vi "Initialise.vi"   [LabVIEW 2020, in "RTAF.lvlib"]
uses:
  RTAF.lvlib
  Actors/Alarms Handler/API/Alarms Handler Actor API.lvclass
  Actors/Logger/API/Logger Actor API.lvclass
  Actors/System Status/API/System Status Actor API.lvclass
  Actors/Test/API/Test Actor API.lvclass
  Actors/Global References.vi
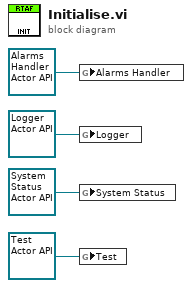
[diagram p0: block diagram]
diagram:
  n1 = global write "Global References.vi" "Alarms Handler"(refnum<class "Alarms Handler Actor API.lvclass"> refnum ("Alarms Handler")) -> ()
  n2 = global write "Global References.vi" "Logger"(refnum<class "Logger Actor API.lvclass"> refnum ("Logger")) -> ()
  n3 = global write "Global References.vi" "System Status"(refnum<class "System Status Actor API.lvclass"> refnum ("System Status")) -> ()
  n4 = global write "Global References.vi" "Test"(refnum<class "Test Actor API.lvclass"> refnum ("Test")) -> ()
